vi "Set Scheme.vi"(8 "error in (no error)":errorcluster, 10 "Scheme":string, 11 "URI in":refnum<class "URI.lvclass">) -> (0 "error out":errorcluster, 3 "URI out":refnum<class "URI.lvclass">)   [LabVIEW 2012, in "Stream.lvlib" / "URI.lvclass"]
uses:
  URI.lvclass
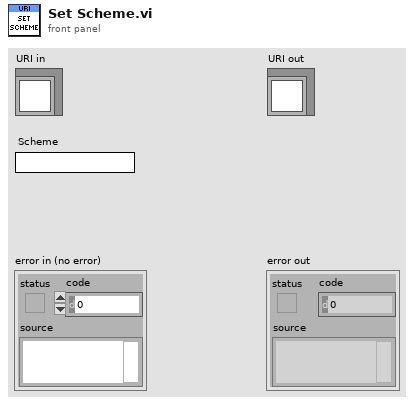
[diagram p1: front panel]
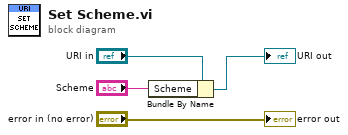
[diagram p0: block diagram]
diagram:
  n1 = Bundle By Name(cluster="URI in", "Scheme"="Scheme") -> (→"URI out":refnum<class "URI.lvclass">)
  "error out" <- "error in (no error)"
